vi "Get String.vi"(8 "error in (no error)":errorcluster, 11 "StringStream in":refnum<class "StringStream.lvclass">) -> (0 "error out":errorcluster, 2 "String":string, 3 "StringStream out":refnum<class "StringStream.lvclass">)   [LabVIEW 2020, in "IO.lvlib" / "StringStream.lvclass"]
uses:
  StringStream.lvclass
  StringStream.lvclass/StringStream.ctl
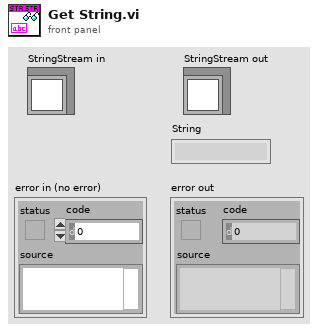
[diagram p1: front panel]
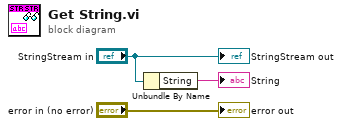
[diagram p0: block diagram]
diagram:
  n1 = Unbundle By Name("StringStream in") -> ("String"=→"String":string)
  "error out" <- "error in (no error)"
  "StringStream out" <- "StringStream in"
